vi "Set sel exp #.vi"(8 "error in (no error)":errorcluster, 10 "Exp sel #":i32, 11 "Control-Client in":refnum<class "Control-Client.lvclass">) -> (0 "error out":errorcluster, 3 "Control-Client out":refnum<class "Control-Client.lvclass">)   [LabVIEW 2015, in "Control-Client.lvclass"]
uses:
  Control-Client.lvclass
  Control-Client.lvclass/Control-Client.ctl
  Experiments/Experiments_group.lvclass/Experiments_group.ctl
  methods/Read Group #.vi
  Experiments/Experiments_group.lvclass
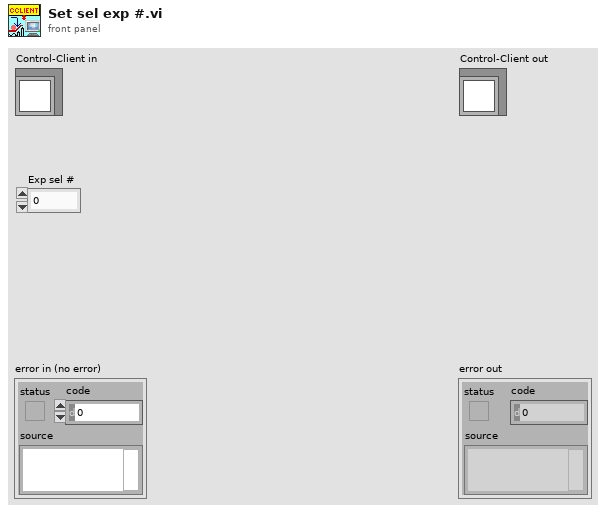
[diagram p1: front panel]
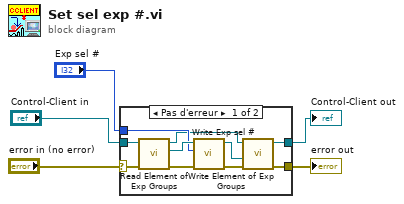
[diagram p0: block diagram]
diagram:
  n1 = case shown="Pas d'erreur" "error in (no error)" {
    selector: "error in (no error)" -> [w14 w17]
    tunnel: [w7 w17] -> w4
    tunnel: [w6 w16] -> w2
    tunnel: "Control-Client in" -> [w15 w16]
    tunnel: "Exp sel #" -> [w12 _]
    frame No Error {
      n2 = call "Read Element of Exp Groups.vi"("error in (no error)"=w14, "Control-Client in"=w15) -> ("error out"=w11:errorcluster, "Experiments_group.lvclass"=w13:refnum<class "Experiments_group.lvclass">, "Control-Client out"=w10:refnum<class "Control-Client.lvclass">)  [unwired: 7 in]
      n3 = call "Write Exp sel #.vi"("error in (no error)"=w11, "Exp sel #"=w12, "Experiments_group in"=w13) -> ("error out"=w8:errorcluster, "Experiments_group out"=w9:refnum<class "Experiments_group.lvclass">)  [unwired: 7 in]
      n4 = call "Write Element of Exp Groups.vi"("error in (no error)"=w8, "Experiments_group.lvclass"=w9, "Control-Client in"=w10) -> ("error out"=w7:errorcluster, "Control-Client out"=w6:refnum<class "Control-Client.lvclass">)  [unwired: 7 in]
    }
    frame Error {
    }
  }
  "error out" <- w4
  "Control-Client out" <- w2
